vi "Monitor Positions + Console.vi"(2 "Array of positions [internal units]":dbl[](array[numeric])=[0.0, 0.0, 0.0, 0.0, 0.0, 0.0, 0.0, 0.0, 0.0, 0.0] caption="Positions [internal units]" step=100.0 format="%#_8f", 7 "refresh rate [ms]":u32=1000 min=50 step=10, 11 "VISA in":refnum<visa-resource-name> caption="VISA in (COM port)") -> ()   [LabVIEW 2011]
doc: "Top-level VI for continuously querying the position of the specified axes."
uses:
  Public/Utility/Axis Name.ctl
  ASI TG-1000.lvlib
panel:
  out "error out update loop":errorcluster
  out "error out event loop":errorcluster
  in  "Move home":bool
  out "Array of status strings":string[](array[string]) caption="Status strings"
  out "Serial response":string
  in  "Send serial command":bool
  in  "Serial command string":string
  in  "Halt movement":bool
  in  "Position step":dbl=100.0
  out "Motors Busy?":bool
  in  "Save Position to File":bool
  in  "Set Position from file":bool
  in  "file path":path
  in  "Array of axes":T1[](array[typedef])=[enum."X", enum."Y", enum."Z", enum."F", enum."undefined", enum."undefined", enum."undefined", enum."undefined", enum."undefined", enum."undefined"]
  in  "Stop program":bool
  # "NB: this VI opens and closes the comm port"
  # "FYI for stages and piezos the internal unit is 0.1um by default"
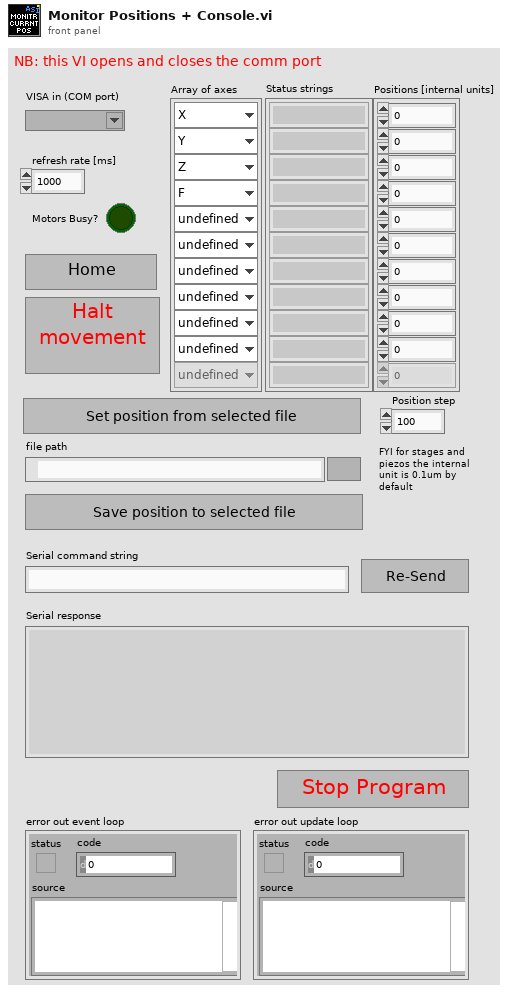
[diagram p1: front panel]
types:
  T1 = typedef "ASI TG-1000.lvlib/Axis Name.ctl" = enum8{"undefined", "A", "B", "C", "D", "E", "F", "G", "H", "I", "J", "K", "L", "M", "N", "O", "P", "Q", "R", "S", "T", "U", "V", "W", "X", "Y", "Z"}
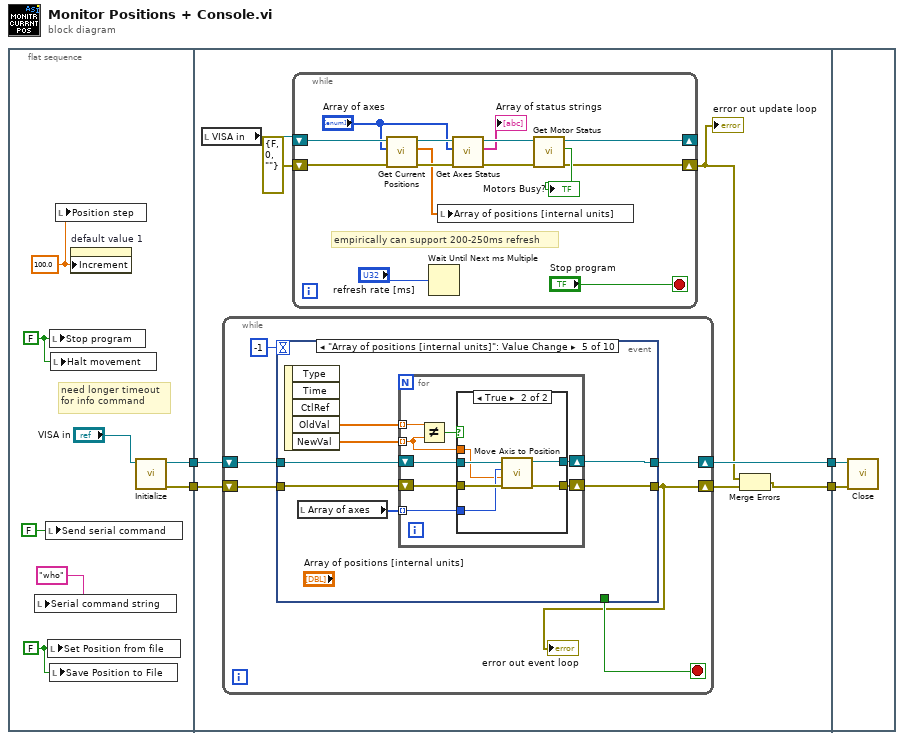
[diagram p0: block diagram]
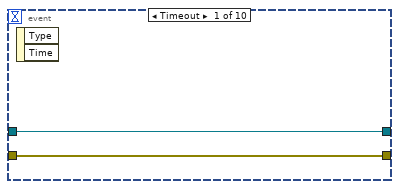
[diagram p2: hidden frame]
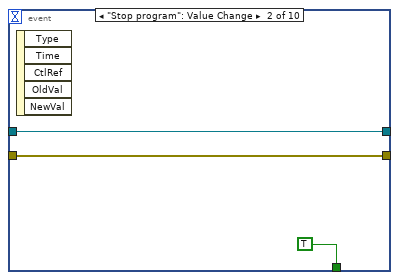
[diagram p3: hidden frame]
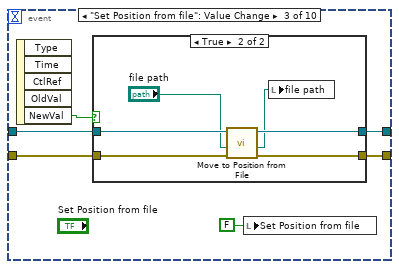
[diagram p4: hidden frame]
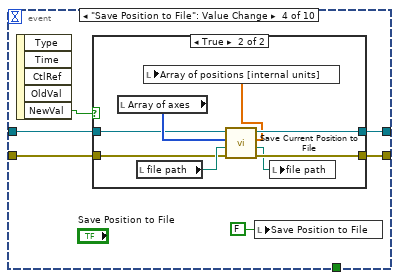
[diagram p6: hidden frame]
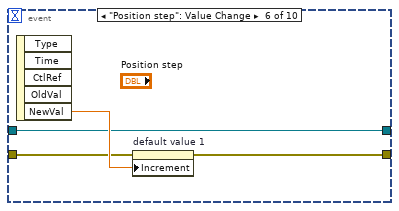
[diagram p9: hidden frame]
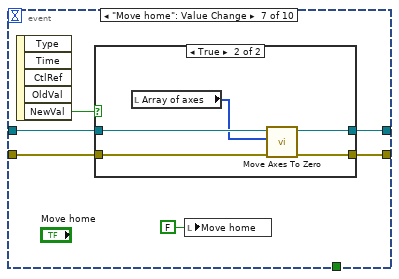
[diagram p10: hidden frame]
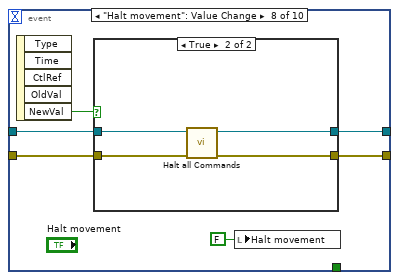
[diagram p12: hidden frame]
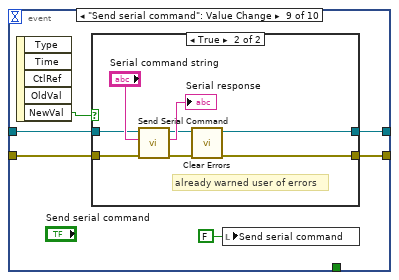
[diagram p14: hidden frame]
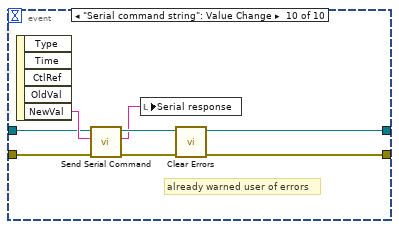
[diagram p16: hidden frame]
diagram:
  n1 = flat-sequence {
    tunnel: [w11] -> w4
    tunnel: [w10] -> w3
    tunnel: w4 -> [w18]
    tunnel: w3 -> [w19]
    tunnel: [w20] -> w2
    tunnel: [w15] -> w1
    tunnel: w2 -> [w151]
    tunnel: w1 -> [w150]
    frame #0 {
      w7 = FALSE ("Set Position from file")
      w5 = 100.0 ("Position inc/dec step")
      w6 = FALSE ("stop")
      # "need longer timeout\nfor info command"
      n2 = local write "Serial command string"("who" ("Serial command string")) -> ()
      n3 = local write "Send serial command"(FALSE ("Send serial command")) -> ()
      n4 = local write "Set Position from file"(w7) -> ()
      n5 = local write "Stop program"(w6) -> ()
      n6 = local write "Save Position to File"(w7) -> ()
      n7 = local write "Halt movement"(w6) -> ()
      n8 = local write "Position step"(w5) -> ()
      n9 = property on="default value 1" class="DigNum (strict)"("Increment"=w5) -> ()  [unwired: 2 in, 2 out]
      n10 = call "Initialize.vi"("VISA resource name"="VISA in") -> ("error out"=w11:errorcluster, "VISA resource name out"=w10:refnum<visa-resource-name>)  [unwired: 9 in]
    }
    frame #1 {
      n11 = local read "VISA in"() -> (w17:refnum<visa-resource-name>)
      n12 = while {
        shift-right: [w39] -> w14
        shift-left: w18 -> [w38]
        shift-right: [w36] -> w20
        shift-left: w19 -> [w37]
        stop <- w40 stop-if-true
        n13 = event shown="[4] \"Array of positions [internal units]\": Value Change" {
          selector: _ -> [_ _ _ _ _ _ _ _ _ _]
          dyn-events: _ -> [_ _ _ _ _ _ _ _ _ _]
          timeout: -1 -> [_ _ _ _ _ _ _ _ _ _]
          tunnel: [_ TRUE _ _ _ _ _ _ _ _] -> w40
          tunnel: [w42 w44 w49 w62 w76 w100 w103 w118 w130 w143] -> w39
          tunnel: w38 -> [w42 w44 w48 w63 w77 w101 w106 w119 w131 w146]
          tunnel: w37 -> [w41 w43 w47 w61 w79 w99 w105 w117 w129 w148]
          tunnel: [w41 w43 w46 w60 w78 w99 w104 w116 w128 w147] -> w36
          event Timeout {
            n14 = event-data() -> ()  [unwired: 1 in, 2 out]
          }
          event "Stop program": Value Change {
            n15 = event-data() -> ()  [unwired: 1 in, 5 out]
          }
          event "Set Position from file": Value Change {
            n16 = event-data() -> ("NewVal"=w51:bool)  [unwired: 1 in, 4 out]
            n17 = case shown="True" w51 {
              tunnel: [w53 w59] -> w49
              tunnel: w48 -> [w53 w58]
              tunnel: w47 -> [w52 w57]
              tunnel: [w52 w56] -> w46
              frame False {
              }
              frame True {
                n18 = call "Move to Position from File.vi"("error in (no error)"=w58, "file path in"="file path", "VISA in"=w57) -> ("error out"=w59:errorcluster, "file path out"=w55:path, "VISA out"=w56:refnum<visa-resource-name>)  [unwired: 6 in]
                n19 = local write "file path"(w55) -> ()
              }
            }
            n20 = local write "Set Position from file"(FALSE ("Set Position from file")) -> ()
          }
          event "Save Position to File": Value Change {
            n21 = event-data() -> ("NewVal"=w65:bool)  [unwired: 1 in, 4 out]
            n22 = case shown="True" w65 {
              tunnel: w63 -> [w67 w73]
              tunnel: [w67 w72] -> w62
              tunnel: w61 -> [w66 w71]
              tunnel: [w66 w70] -> w60
              frame False {
              }
              frame True {
                n23 = local read "Array of axes"() -> (w74:T1[])
                n24 = local read "file path"() -> (w75:path)
                n25 = call "Save Current Position to File.vi"("error in (no error)"=w73, "file path"=w75, "Array of axes"=w74, "VISA in"=w71) -> ("error out"=w72:errorcluster, "file path out"=w69:path, "Array of positions [um]"=w68:dbl[], "VISA out"=w70:refnum<visa-resource-name>)  [unwired: 4 in]
                n26 = local write "Array of positions [internal units]"(w68) -> ()
                n27 = local write "file path"(w69) -> ()
              }
            }
            n28 = local write "Save Position to File"(FALSE ("Save Position to File")) -> ()
          }
          event "Array of positions [internal units]": Value Change {
            n29 = event-data() -> ("OldVal"=w82:dbl[], "NewVal"=w81:dbl[])  [unwired: 1 in, 3 out]
            n30 = local read "Array of axes"() -> (w80:T1[])
            n31 = for {
              tunnel: w82 -> [w90] mode=indexing
              tunnel: w81 -> [w83] mode=indexing
              tunnel: w80 -> [w84] mode=indexing
              shift-right: [w85] -> w76
              shift-left: w77 -> [w86]
              shift-right: [w87] -> w78
              shift-left: w79 -> [w88]
              n32 = Not Equal?(x=w90, y=w83) -> (x != y?=w89:bool)
              n33 = case shown="True" w89 {
                tunnel: w88 -> [w92 w98]
                tunnel: [w92 w97] -> w87
                tunnel: w86 -> [w91 w96]
                tunnel: [w91 w95] -> w85
                tunnel: w84 -> [_ w94]
                tunnel: w83 -> [_ w93]
                frame False {
                }
                frame True {
                  n34 = call "Move Axis to Position.vi"("error in (no error)"=w96, "Position [internal units]"=w93, "Axis"=w94, "VISA in"=w98) -> ("error out"=w95:errorcluster, "VISA out"=w97:refnum<visa-resource-name>)  [unwired: 5 in]
                }
              }
            }
          }
          event "Position step": Value Change {
            n35 = event-data() -> ("NewVal"=w102:dbl)  [unwired: 1 in, 4 out]
            n36 = property on="default value 1" class="DigNum (strict)"(error in=w101, "Increment"=w102) -> (error out=w100:errorcluster)  [unwired: 1 in, 1 out]
          }
          event "Move home": Value Change {
            n37 = event-data() -> ("NewVal"=w108:bool)  [unwired: 1 in, 4 out]
            n38 = case shown="True" w108 {
              tunnel: w106 -> [w109 w112]
              tunnel: w105 -> [w110 w115]
              tunnel: [w110 w114] -> w104
              tunnel: [w109 w113] -> w103
              frame False {
              }
              frame True {
                n39 = local read "Array of axes"() -> (w111:T1[])
                n40 = call "Move Axes To Zero.vi"("error in (no error)"=w112, "Array of axes"=w111, "VISA in"=w115) -> ("error out"=w113:errorcluster, "VISA out"=w114:refnum<visa-resource-name>)  [unwired: 6 in]
              }
            }
            n41 = local write "Move home"(FALSE ("Move home")) -> ()
          }
          event "Halt movement": Value Change {
            n42 = event-data() -> ("NewVal"=w121:bool)  [unwired: 1 in, 4 out]
            n43 = case shown="True" w121 {
              tunnel: w119 -> [w123 w127]
              tunnel: [w123 w126] -> w118
              tunnel: w117 -> [w122 w125]
              tunnel: [w122 w124] -> w116
              frame False {
              }
              frame True {
                n44 = call "Halt all Commands.vi"("error in (no error)"=w127, "VISA in"=w125) -> ("error out"=w126:errorcluster, "VISA out"=w124:refnum<visa-resource-name>)  [unwired: 7 in]
              }
            }
            n45 = local write "Halt movement"(FALSE ("Halt movement")) -> ()
          }
          event "Send serial command": Value Change {
            n46 = event-data() -> ("NewVal"=w132:bool)  [unwired: 1 in, 4 out]
            n47 = case shown="True" w132 {
              tunnel: w131 -> [w135 w141]
              tunnel: [w135 w136] -> w130
              tunnel: w129 -> [w134 w138]
              tunnel: [w134 w137] -> w128
              frame False {
              }
              frame True {
                # "already warned user of errors"
                n48 = call "Send Serial Command.vi"("error in (no error)"=w141, "Command"="Serial command string", "VISA in"=w138) -> ("error out"=w140:errorcluster, "Response"=→"Serial response":string, "VISA out"=w137:refnum<visa-resource-name>)  [unwired: 6 in]
                n49 = call <vilib>:"Clear Errors.vi"("error in (no error)"=w140) -> ("error out"=w136:errorcluster)  [unwired: 6 in]
              }
            }
            n50 = local write "Send serial command"(FALSE ("Send serial command")) -> ()
          }
          event "Serial command string": Value Change {
            # "already warned user of errors"
            n51 = event-data() -> ("NewVal"=w149:string)  [unwired: 1 in, 4 out]
            n52 = call "Send Serial Command.vi"("error in (no error)"=w146, "Command"=w149, "VISA in"=w148) -> ("error out"=w145:errorcluster, "Response"=w144:string, "VISA out"=w147:refnum<visa-resource-name>)  [unwired: 6 in]
            n53 = local write "Serial response"(w144) -> ()
            n54 = call <vilib>:"Clear Errors.vi"("error in (no error)"=w145) -> ("error out"=w143:errorcluster)  [unwired: 6 in]
          }
        }
        "error out event loop" <- w39
      }
      n55 = while {
        shift-right: [w24] -> _
        shift-left: w17 -> [w26]
        shift-right: [w23] -> w13
        shift-left: errorcluster {"status"=FALSE, "code"=0, "source"=""} ("error out") -> [w25]
        stop <- "Stop program" stop-if-true
        # "empirically can support 200-250ms refresh"
        n56 = call "Get Current Positions.vi"("error in (no error)"=w25, "Array of axes"="Array of axes", "VISA in"=w26) -> ("error out"=w32:errorcluster, "Array of positions [internal units]"=w21:dbl[], "VISA out"=w33:refnum<visa-resource-name>)  [unwired: 6 in]
        n57 = Wait Until Next ms Multiple(millisecond multiple="refresh rate [ms]") -> ()  [unwired: 1 out]
        n58 = local write "Array of positions [internal units]"(w21) -> ()
        n59 = call "Get Axes Status.vi"("error in (no error)"=w32, "Array of axes"="Array of axes", "VISA in"=w33) -> ("error out"=w31:errorcluster, "Array of status strings"=→"Array of status strings":string[], "VISA out"=w30:refnum<visa-resource-name>)  [unwired: 6 in]
        n60 = call "Get Motor Status.vi"("error in (no error)"=w31, "VISA in"=w30) -> ("error out"=w23:errorcluster, "Motors Busy?"=→"Motors Busy?":bool, "VISA out"=w24:refnum<visa-resource-name>)  [unwired: 6 in]
      }
      "error out update loop" <- w13
      n61 = Merge Errors(w13, w14) -> (w15:errorcluster)
    }
    frame #2 {
      n62 = call "Close.vi"("error in (no error)"=w150, "VISA resource name"=w151) -> ()  [unwired: 9 in, 1 out]
    }
  }
